vi "StringArray2InfoOfPlayerCluster.vi"(1 "数组":string[](array[string])) -> (0 "玩家信息":T1)   [LabVIEW 2019]
uses:
  ctl/InfoOfPlayer.ctl
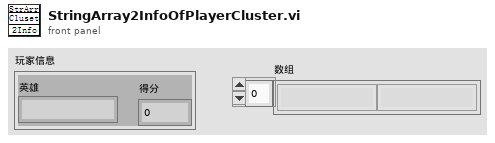
[diagram p1: front panel]
types:
  T1 = typedef "InfoOfPlayer.ctl" = cluster{"得分":i32, "英雄":string}
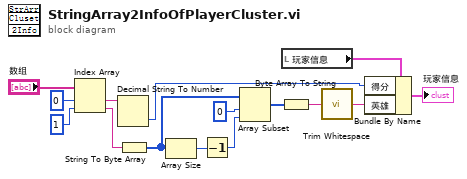
[diagram p0: block diagram]
diagram:
  n1 = Index Array(array="数组", index #1=0 ("索引"), index #2=1 ("索引")) -> (element #1=w10:string, element #2=w5:string)
  n2 = Decimal String To Number(string=w10) -> (number=w9:i32)  [unwired: 2 in, 1 out]
  n3 = String To Byte Array(string=w5) -> (unsigned byte array=w4:u8[])
  n4 = Array Size(array=w4) -> (size(s)=w8:i32)
  n5 = Decrement(x=w8) -> (x-1=w6:i32)
  n6 = Array Subset(array=w4, index=0 ("索引"), length=w6) -> (w3:u8[])
  n7 = Byte Array To String(unsigned byte array=w3) -> (string=w2:string)
  n8 = local read "玩家信息"() -> (w12:T1)
  n9 = call <vilib>:"Trim Whitespace.vi"("string"=w2) -> ("trimmed string"=w1:string)  [unwired: 1 in]
  n10 = Bundle By Name(cluster=w12, "得分"=w9, "英雄"=w1) -> (→"玩家信息":T1)
